vi "VI Scripting Open Path From VI.vi"(11 "Path":path) -> (0 "Reverse Path?":bool, 1 "path":cluster{"X":dbl, "Y":dbl}[](array[cluster]), 2 "Data Points":T1[](array[typedef]), 3 "Graph":cluster{dbl[], dbl[]}[](array[cluster]), 5 "Name":string)   [LabVIEW 2018]
uses:
  Typedef/Data Point.ctl
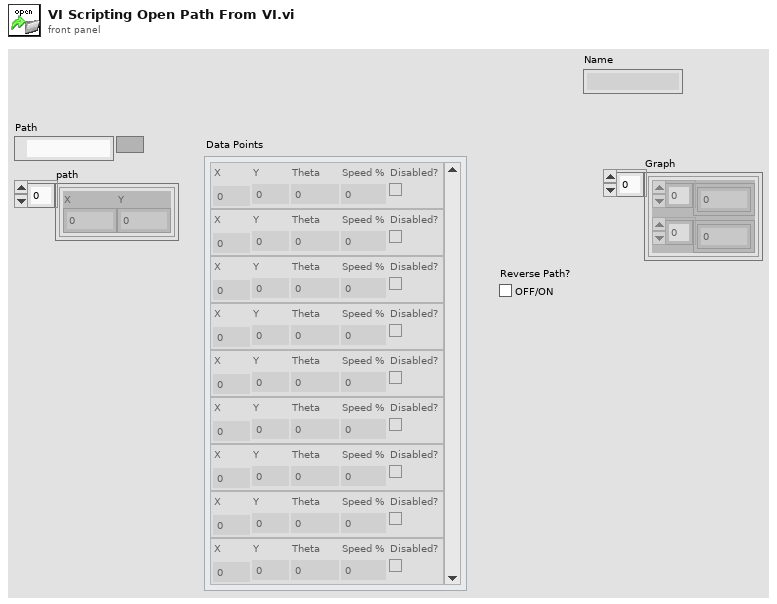
[diagram p1: front panel]
types:
  T1 = typedef "Data Point.ctl" = cluster{"X":dbl, "Y":dbl, "Theta":dbl, "Speed %":dbl, "Disabled?":bool}
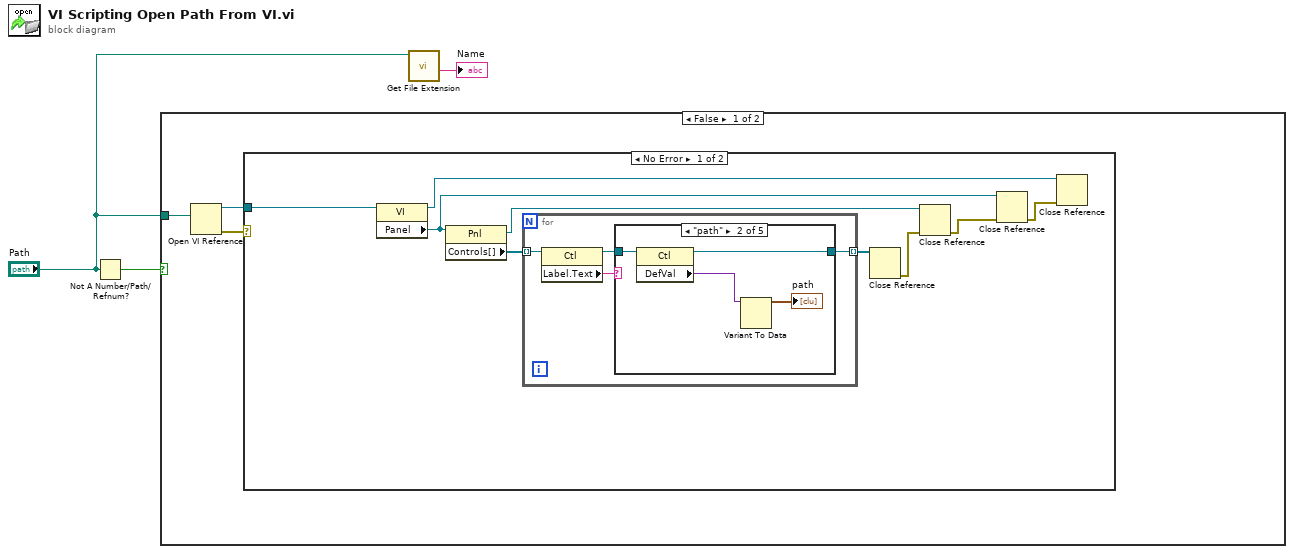
[diagram p0: block diagram]
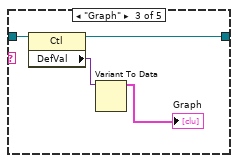
[diagram p3: hidden frame]
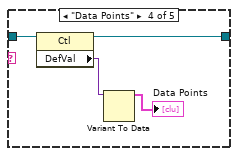
[diagram p4: hidden frame]
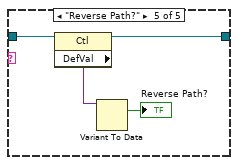
[diagram p5: hidden frame]
diagram:
  n1 = Not A Number/Path/Refnum?(number/path/refnum="Path") -> (NaN/Path/Refnum?=w3:bool)
  n2 = case shown="False" w3 {
    tunnel: "Path" -> [w6 _]
    frame False {
      n3 = Open VI Reference(vi path=w6) -> (vi reference=w4:refnum<vi>, error out=w5:errorcluster)  [unwired: 5 in]
      n4 = case shown="No Error" w5 {
        tunnel: w4 -> [w9 _]
        frame No Error {
          n5 = property class="VI"(reference=w9) -> (reference out=w7:refnum<vi>, "Panel"=w10:refnum<vi>)  [unwired: 1 in, 1 out]
          n6 = property class="Pnl"(reference=w10) -> (reference out=w15:refnum<vi>, "Controls[]"=w12:refnum<vi>[])  [unwired: 1 in, 1 out]
          n7 = for {
            tunnel: w12 -> [w19] mode=indexing
            tunnel: [w16] -> w13 mode=indexing
            n8 = property class="Ctl"(reference=w19) -> (reference out=w17:refnum<vi>, "Label.Text"=w18:string)  [unwired: 1 in, 1 out]
            n9 = case shown="\"path\"" w18 {
              tunnel: w17 -> [w20 w24 w28 w32 w36]
              tunnel: [w20 w23 w27 w31 w35] -> w16
              frame Default {
              }
              frame "path" {
                n10 = property class="Ctl"(reference=w24) -> (reference out=w23:refnum<vi>, "DefVal"=w22:variant)  [unwired: 1 in, 1 out]
                n11 = Variant To Data(Variant=w22) -> (data=→"path":cluster{"X":dbl, "Y":dbl}[])  [unwired: 2 in, 1 out]
              }
              frame "Graph" {
                n12 = property class="Ctl"(reference=w28) -> (reference out=w27:refnum<vi>, "DefVal"=w26:variant)  [unwired: 1 in, 1 out]
                n13 = Variant To Data(Variant=w26) -> (data=→"Graph":cluster{dbl[], dbl[]}[])  [unwired: 2 in, 1 out]
              }
              frame "Data Points" {
                n14 = property class="Ctl"(reference=w32) -> (reference out=w31:refnum<vi>, "DefVal"=w30:variant)  [unwired: 1 in, 1 out]
                n15 = Variant To Data(Variant=w30) -> (data=→"Data Points":T1[])  [unwired: 2 in, 1 out]
              }
              frame "Reverse Path?" {
                n16 = property class="Ctl"(reference=w36) -> (reference out=w35:refnum<vi>, "DefVal"=w33:variant)  [unwired: 1 in, 1 out]
                n17 = Variant To Data(Variant=w33) -> (data=→"Reverse Path?":bool)  [unwired: 2 in, 1 out]
              }
            }
          }
          n18 = Close Reference(reference=w13) -> (error out=w14:errorcluster)  [unwired: 1 in]
          n19 = Close Reference(reference=w15, error in (no error)=w14) -> (error out=w11:errorcluster)
          n20 = Close Reference(reference=w10, error in (no error)=w11) -> (error out=w8:errorcluster)
          n21 = Close Reference(reference=w7, error in (no error)=w8) -> ()  [unwired: 1 out]
        }
        frame Error {
        }
      }
    }
    frame True {
    }
  }
  n22 = call <vilib>:"Get File Extension.vi"("file"="Path") -> ("filename without extension"=→"Name":string)  [unwired: 6 in, 4 out]
